vi "Configure Acquisition.vi"(8 "Error In":errorcluster, 11 "eCRDS in":refnum<class "eCRDS.lvclass">) -> (0 "error out":errorcluster, 3 "eCRDS out":refnum<class "eCRDS.lvclass">)   [LabVIEW 2014, in "eCRDS Library.lvlib" / "eCRDS.lvclass"]
doc: "Configure the blue channel for generation and acquisition of the laser signal. The acquisition of the laser signal is run off of a retriggerable clock signal that operates in bursts. When the clock runs, a signal is acquired. The clock only runs when the digital output for the laser goes high. It then generates a finite number of signals until the laser output goes high again.\n\nThe clock for the AI runs off of the same board as the AI. The clock is triggered via a signal run across the backplane on PXI_Trig0 that is connected to the generation signal on the housekeeping card."
uses:
  eCRDS.lvclass
  eCRDS.lvclass/eCRDS.ctl
  reusable/Instrument/Instrument.lvclass/Instrument.ctl
  reusable/Instrument/Read Log Session.vi
  <vilib>/DAQmx/configure/timing.llb/DAQmx Timing (Implicit).vi
  <vilib>/DAQmx/configure/timing.llb/DAQmx Timing (Sample Clock).vi
  <userlib>/_Session Fwk/Session - Root.lvclass
  <resource>/objmgr/daqmx.rc
  <vilib>/DAQmx/configure/trigger.llb/DAQmx Start Trigger (Digital Edge).vi
  reusable/Session APIs/Session Log/System Log.lvclass
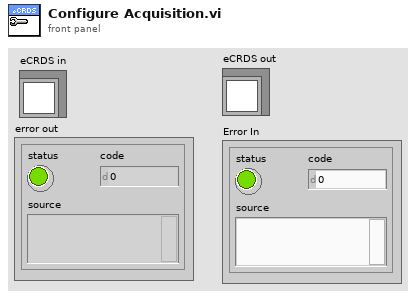
[diagram p1: front panel]
types:
  T1 = typedef "Session - Root.lvclass/Session Handle.ctl" = refnum<data-value>
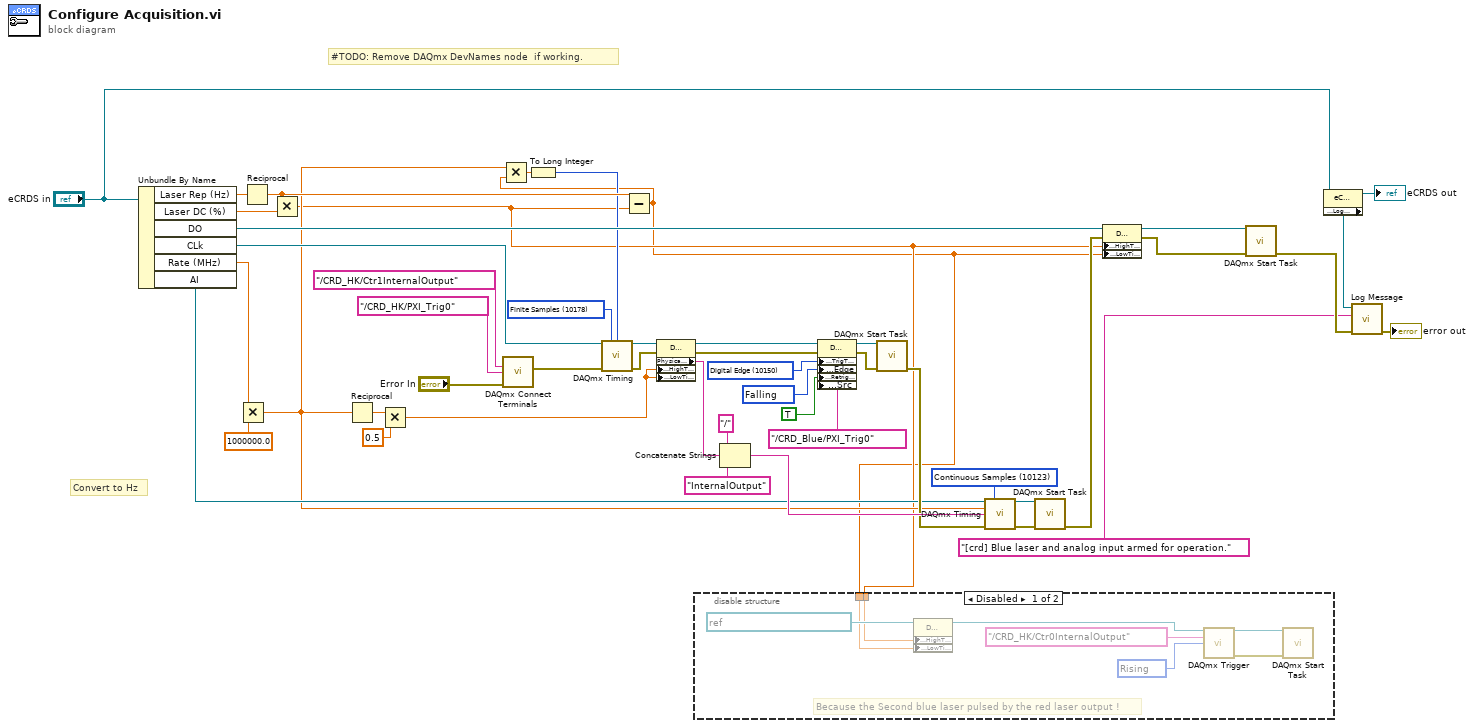
[diagram p0: block diagram]
diagram:
  w48 = 10123 items=["Finite Samples"=10178, "Continuous Samples"=10123, "Hardware Timed Single Point"=12522] ("sample mode")
  w39 = 10171 items=["Rising"=10280, "Falling"=10171] ("Ref.DigEdge.Edge")
  w38 = 10150 items=["Analog Edge"=10099, "Digital Edge"=10150, "Digital Pattern"=10398, "Analog Window"=10103, "None"=10230] ("Ref.TrigType")
  w31 = 10178 items=["Finite Samples"=10178, "Continuous Samples"=10123, "Hardware Timed Single Point"=12522] ("sample mode")
  # "#TODO: Remove DAQmx DevNames node  if working."
  # "Convert to Hz"
  n1 = Unbundle By Name("eCRDS in") -> ("Laser Rep (Hz)"=w5:dbl, "Laser DC (%)"=w6:dbl, "DO"=w17:refnum<k21>, "CLk"=w24:refnum<k21>, "Rate (MHz)"=w10:dbl, "AI"=w15:refnum<k21>)
  n2 = Multiply(x=w10, y=1000000.0) -> (x*y=w9:dbl)
  n3 = Reciprocal(x=w5) -> (1/x=w11:dbl)
  n4 = Multiply(x=w11, y=w6) -> (x*y=w4:dbl)
  n5 = Reciprocal(x=w9) -> (1/x=w14:dbl)
  n6 = Multiply(x=w14, y=0.5) -> (x*y=w12:dbl)
  n7 = call <vilib>:"DAQmx Connect Terminals.vi"("source terminal"=tag "/CRD_HK/Ctr1InternalOutput", "destination terminal"=tag "/CRD_HK/PXI_Trig0", "error in"="Error In") -> ("error out"=w25:errorcluster)  [unwired: 12 in]
  n8 = Subtract(x=w11, y=w4) -> (x-y=w3:dbl)
  n9 = Multiply(x=w9, y=w3) -> (x*y=w8:dbl)
  n10 = To Long Integer(number=w8) -> (32bit integer=w7:i32)
  n11 = call-poly <vilib>:"DAQmx Timing.vi"("task/channels in"=w24, "sample mode"=w31, "samples per channel"=w7, "error in"=w25) -> ("task out"=w32:refnum<k21>, "error out"=w41:errorcluster)  [unwired: 10 in]
  n12 = property class="DAQmx Channel"(reference=w32, error in=w41, "CO.Pulse.HighTime"=w12, "CO.Pulse.LowTime"=w12) -> (reference out=w37:refnum<k21>, error out=w42:errorcluster, "PhysicalChanName"=w35:tag)
  n13 = disable-structure shown="Disabled" {
    disable-tunnel: w4 -> [w51 _]
    disable-tunnel: w3 -> [w50 _]
    frame Disabled {
      w53 = 10280 items=["Rising"=10280, "Falling"=10171] ("edge")
      # "Because the Second blue laser pulsed by the red laser output !"
      n14 = property class="DAQmx Channel"(reference=refnum<k21> "CRD Red Laser Output" ("task"), "CO.Pulse.HighTime"=w51, "CO.Pulse.LowTime"=w50) -> (reference out=w55:refnum<k21>)  [unwired: 1 in, 1 out]
      n15 = call-poly <vilib>:"DAQmx Trigger.vi"("task/channels in"=w55, "source"=tag "/CRD_HK/Ctr0InternalOutput" ("source terminal"), "edge"=w53) -> ("task out"=w52:refnum<k21>, "error out"=w49:errorcluster)  [unwired: 11 in]
      n16 = call <vilib>:"DAQmx Start Task.vi"("task/channels in"=w52, "error in"=w49) -> ()  [unwired: 12 in, 2 out]
    }
    frame Enabled {
    }
  }
  n17 = Concatenate Strings("/" ("string"), w35, "InternalOutput" ("string")) -> (w36:string)
  n18 = property class="DAQmx Trigger"(reference=w37, error in=w42, "Start.TrigType"=w38, "Start.DigEdge.Edge"=w39, "Start.Retriggerable"=TRUE, "Start.DigEdge.Src"=tag "/CRD_Blue/PXI_Trig0") -> (reference out=w43:refnum<k21>, error out=w44:errorcluster)
  n19 = call <vilib>:"DAQmx Start Task.vi"("task/channels in"=w43, "error in"=w44) -> ("error out"=w30:errorcluster)  [unwired: 12 in, 1 out]
  n20 = call-poly <vilib>:"DAQmx Timing.vi"("task/channels in"=w15, "sample mode"=w48, "rate"=w9, "source"=w36, "error in"=w30) -> ("task out"=w45:refnum<k21>, "error out"=w46:errorcluster)  [unwired: 9 in]
  n21 = call <vilib>:"DAQmx Start Task.vi"("task/channels in"=w45, "error in"=w46) -> ("error out"=w16:errorcluster)  [unwired: 12 in, 1 out]
  n22 = property class="DAQmx Channel"(reference=w17, error in=w16, "CO.Pulse.HighTime"=w4, "CO.Pulse.LowTime"=w3) -> (reference out=w2:refnum<k21>, error out=w1:errorcluster)
  n23 = call <vilib>:"DAQmx Start Task.vi"("task/channels in"=w2, "error in"=w1) -> ("error out"=w20:errorcluster)  [unwired: 12 in, 1 out]
  n24 = property class="eCRDS"(reference="eCRDS in") -> (reference out=→"eCRDS out":refnum<class "eCRDS.lvclass">, "Accessors:Log Session"=w26:T1)  [unwired: 1 in, 1 out]
  n25 = call "Log Message.vi"("error in"=w20, "MSG In"="[crd] Blue laser and analog input armed for operation.", "session in"=w26) -> ("error out"=→"error out":errorcluster)  [unwired: 7 in, 1 out]
